vi "checkError.vi"(3 "error in":errorcluster) -> (0 "Time out":bool, 1 "error out":errorcluster)   [LabVIEW 2011]
doc: "Description:\n\nThis vi checks if there is an timeout-error present."
panel:
  in  "clean error in":errorcluster
  in  "clean error in":errorcluster
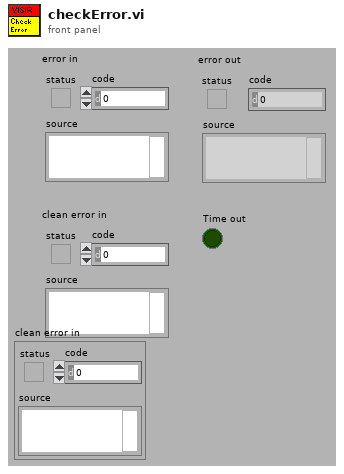
[diagram p1: front panel]
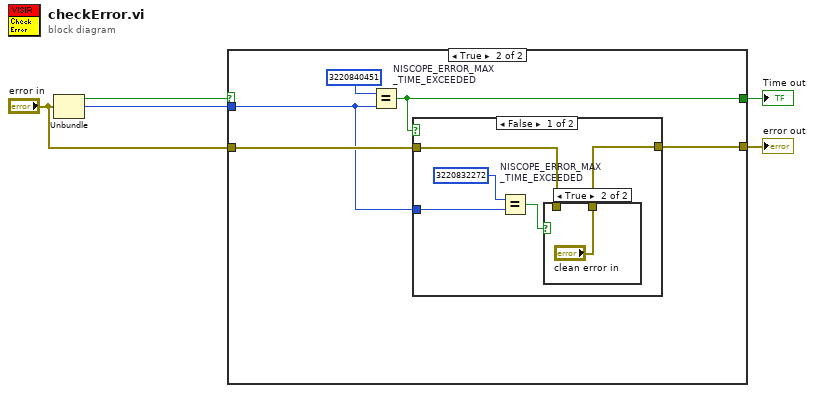
[diagram p0: block diagram]
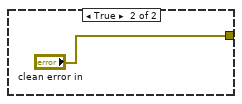
[diagram p4: hidden frame]
diagram:
  n1 = Unbundle("error in") -> ("status"=w5:bool, "code"=w4:i32)  [unwired: 1 out]
  n2 = case shown="True" w5 {
    selector: w5 -> [w6 _]
    tunnel: w4 -> [_ w8]
    tunnel: [w6 w12] -> w3
    tunnel: [w7 w10] -> w2
    tunnel: "error in" -> [w7 w9]
    frame False {
    }
    frame True {
      w11 = u32 3220840451  # NISCOPE_ERROR_MAX _TIME_EXCEEDED
      n3 = Equal?(x=w11, y=w8) -> (x = y?=w12:bool)
      n4 = case shown="False" w12 {
        tunnel: [w14 "clean error in"] -> w10
        tunnel: w9 -> [w13 _]
        tunnel: w8 -> [w15 _]
        frame False {
          w17 = u32 3220832272  # NISCOPE_ERROR_MAX _TIME_EXCEEDED
          n5 = Equal?(x=w17, y=w15) -> (x = y?=w16:bool)
          n6 = case shown="True" w16 {
            tunnel: [w18 "clean error in"] -> w14
            tunnel: w13 -> [w18 _]
            frame False {
            }
            frame True {
            }
          }
        }
        frame True {
        }
      }
    }
  }
  "Time out" <- w3
  "error out" <- w2
